vi "Digital_Bridge_3_kart.vi"() -> ()   [LabVIEW 2014] (continued)
                                n4059 = Index Array(array=w2316, index (row)=w2315, index (col)=w2314) -> (element=w2313:dbl)
                                n4060 = Replace Array Subset(array=w2316, new element=w2313, index (row)=w2315, index (col)=w2314) -> (w2317:dbl[][])
                                }
                                }
                                n4061 = local write "Denge Kosulu x2_y2"(w2257) -> ()
                                }
                              }
                              frame 3 {
                                n4062 = for {
                                N: 10 -> [_]
                                tunnel: w2318 -> [w2320]
                                i -> [w2323]
                                n4063 = local read "Denge Kosulu x2_y2"() -> (w2322:dbl[][])
                                n4064 = case shown="6" w2323 {
                                tunnel: w2323 -> [w2325 w2330 w2337 w2344 w2351 w2358 w2366 w2371 w2374 w2379]
                                tunnel: w2322 -> [w2326 w2332 w2336 w2343 w2350 w2357 w2364 w2369 w2375 w2380]
                                tunnel: [w2327 w2333 w2334 w2342 w2349 w2356 w2363 w2368 w2376 w2381] -> w2321
                                tunnel: w2320 -> [w2328 w2331 w2335 w2341 w2348 w2355 w2365 w2370 w2373 w2378]
                                frame 0, Default {
                                n4065 = Index Array(array=w2326, index (row)=w2325, index (col)=w2328) -> (element=w2324:dbl)
                                n4066 = Replace Array Subset(array=w2326, new element=w2324, index (row)=w2325, index (col)=w2328) -> (w2327:dbl[][])
                                }
                                frame 1 {
                                n4067 = Index Array(array=w2332, index (row)=w2330, index (col)=w2331) -> (element=w2329:dbl)
                                n4068 = Replace Array Subset(array=w2332, new element=w2329, index (row)=w2330, index (col)=w2331) -> (w2333:dbl[][])
                                }
                                frame 2 {
                                n4069 = Index Array(array=w2336, index (row)=w2337, index (col)=w2335) -> (element=w2340:dbl)
                                n4070 = Multiply(x=w2340, y=2.0) -> (x*y=w2338:dbl)
                                n4071 = Replace Array Subset(array=w2336, new element=w2338, index (row)=w2337, index (col)=w2335) -> (w2334:dbl[][])
                                }
                                frame 3 {
                                n4072 = Index Array(array=w2343, index (row)=w2344, index (col)=w2341) -> (element=w2347:dbl)
                                n4073 = Multiply(x=w2347, y=2.0) -> (x*y=w2345:dbl)
                                n4074 = Replace Array Subset(array=w2343, new element=w2345, index (row)=w2344, index (col)=w2341) -> (w2342:dbl[][])
                                }
                                frame 4 {
                                n4075 = Index Array(array=w2350, index (row)=w2351, index (col)=w2348) -> (element=w2354:dbl)
                                n4076 = Multiply(x=w2354, y=2.0) -> (x*y=w2352:dbl)
                                n4077 = Replace Array Subset(array=w2350, new element=w2352, index (row)=w2351, index (col)=w2348) -> (w2349:dbl[][])
                                }
                                frame 5 {
                                n4078 = Index Array(array=w2357, index (row)=w2358, index (col)=w2355) -> (element=w2361:dbl)
                                n4079 = Multiply(x=w2361, y=2.0) -> (x*y=w2359:dbl)
                                n4080 = Replace Array Subset(array=w2357, new element=w2359, index (row)=w2358, index (col)=w2355) -> (w2356:dbl[][])
                                }
                                frame 6 {
                                n4081 = Index Array(array=w2364, index (row)=w2366, index (col)=w2365) -> (element=w2362:dbl)
                                n4082 = Replace Array Subset(array=w2364, new element=w2362, index (row)=w2366, index (col)=w2365) -> (w2363:dbl[][])
                                }
                                frame 7 {
                                n4083 = Index Array(array=w2369, index (row)=w2371, index (col)=w2370) -> (element=w2367:dbl)
                                n4084 = Replace Array Subset(array=w2369, new element=w2367, index (row)=w2371, index (col)=w2370) -> (w2368:dbl[][])
                                }
                                frame 8 {
                                n4085 = Index Array(array=w2375, index (row)=w2374, index (col)=w2373) -> (element=w2372:dbl)
                                n4086 = Replace Array Subset(array=w2375, new element=w2372, index (row)=w2374, index (col)=w2373) -> (w2376:dbl[][])
                                }
                                frame 9 {
                                n4087 = Index Array(array=w2380, index (row)=w2379, index (col)=w2378) -> (element=w2377:dbl)
                                n4088 = Replace Array Subset(array=w2380, new element=w2377, index (row)=w2379, index (col)=w2378) -> (w2381:dbl[][])
                                }
                                }
                                n4089 = local write "Denge Kosulu x2_y2"(w2321) -> ()
                                }
                              }
                              frame 4, Default {
                                n4090 = for {
                                N: 10 -> [_]
                                tunnel: w2382 -> [w2384]
                                i -> [w2387]
                                n4091 = local read "Denge Kosulu x2_y2"() -> (w2386:dbl[][])
                                n4092 = case shown="6" w2387 {
                                tunnel: w2387 -> [w2389 w2394 w2402 w2407 w2412 w2417 w2421 w2428 w2434 w2439]
                                tunnel: w2386 -> [w2390 w2396 w2401 w2406 w2411 w2416 w2419 w2426 w2435 w2440]
                                tunnel: [w2391 w2397 w2399 w2405 w2410 w2415 w2418 w2425 w2436 w2441] -> w2385
                                tunnel: w2384 -> [w2392 w2395 w2400 w2404 w2409 w2414 w2420 w2427 w2433 w2438]
                                frame 0, Default {
                                n4093 = Index Array(array=w2390, index (row)=w2389, index (col)=w2392) -> (element=w2388:dbl)
                                n4094 = Replace Array Subset(array=w2390, new element=w2388, index (row)=w2389, index (col)=w2392) -> (w2391:dbl[][])
                                }
                                frame 1 {
                                n4095 = Index Array(array=w2396, index (row)=w2394, index (col)=w2395) -> (element=w2393:dbl)
                                n4096 = Replace Array Subset(array=w2396, new element=w2393, index (row)=w2394, index (col)=w2395) -> (w2397:dbl[][])
                                }
                                frame 2 {
                                n4097 = Index Array(array=w2401, index (row)=w2402, index (col)=w2400) -> (element=w2398:dbl)
                                n4098 = Replace Array Subset(array=w2401, new element=w2398, index (row)=w2402, index (col)=w2400) -> (w2399:dbl[][])
                                }
                                frame 3 {
                                n4099 = Index Array(array=w2406, index (row)=w2407, index (col)=w2404) -> (element=w2403:dbl)
                                n4100 = Replace Array Subset(array=w2406, new element=w2403, index (row)=w2407, index (col)=w2404) -> (w2405:dbl[][])
                                }
                                frame 4 {
                                n4101 = Index Array(array=w2411, index (row)=w2412, index (col)=w2409) -> (element=w2408:dbl)
                                n4102 = Replace Array Subset(array=w2411, new element=w2408, index (row)=w2412, index (col)=w2409) -> (w2410:dbl[][])
                                }
                                frame 5 {
                                n4103 = Index Array(array=w2416, index (row)=w2417, index (col)=w2414) -> (element=w2413:dbl)
                                n4104 = Replace Array Subset(array=w2416, new element=w2413, index (row)=w2417, index (col)=w2414) -> (w2415:dbl[][])
                                }
                                frame 6 {
                                n4105 = Index Array(array=w2419, index (row)=w2421, index (col)=w2420) -> (element=w2424:dbl)
                                n4106 = Multiply(x=w2424, y=2.0) -> (x*y=w2422:dbl)
                                n4107 = Replace Array Subset(array=w2419, new element=w2422, index (row)=w2421, index (col)=w2420) -> (w2418:dbl[][])
                                }
                                frame 7 {
                                n4108 = Index Array(array=w2426, index (row)=w2428, index (col)=w2427) -> (element=w2431:dbl)
                                n4109 = Multiply(x=w2431, y=2.0) -> (x*y=w2429:dbl)
                                n4110 = Replace Array Subset(array=w2426, new element=w2429, index (row)=w2428, index (col)=w2427) -> (w2425:dbl[][])
                                }
                                frame 8 {
                                n4111 = Index Array(array=w2435, index (row)=w2434, index (col)=w2433) -> (element=w2432:dbl)
                                n4112 = Replace Array Subset(array=w2435, new element=w2432, index (row)=w2434, index (col)=w2433) -> (w2436:dbl[][])
                                }
                                frame 9 {
                                n4113 = Index Array(array=w2440, index (row)=w2439, index (col)=w2438) -> (element=w2437:dbl)
                                n4114 = Replace Array Subset(array=w2440, new element=w2437, index (row)=w2439, index (col)=w2438) -> (w2441:dbl[][])
                                }
                                }
                                n4115 = local write "Denge Kosulu x2_y2"(w2385) -> ()
                                }
                              }
                              frame 5 {
                                n4116 = for {
                                N: 10 -> [_]
                                tunnel: w2442 -> [w2444]
                                i -> [w2447]
                                n4117 = local read "Denge Kosulu x2_y2"() -> (w2446:dbl[][])
                                n4118 = case shown="6" w2447 {
                                tunnel: w2447 -> [w2448 w2455 w2466 w2471 w2476 w2481 w2486 w2491 w2496 w2500]
                                tunnel: w2446 -> [w2449 w2457 w2465 w2470 w2475 w2480 w2484 w2489 w2497 w2501]
                                tunnel: [w2450 w2458 w2463 w2469 w2474 w2479 w2483 w2488 w2498 w2502] -> w2445
                                tunnel: w2444 -> [w2451 w2456 w2464 w2468 w2473 w2478 w2485 w2490 w2495 w2499]
                                frame 0, Default {
                                n4119 = Index Array(array=w2449, index (row)=w2448, index (col)=w2451) -> (element=w2454:dbl)
                                n4120 = Multiply(x=w2454, y=2.0) -> (x*y=w2452:dbl)
                                n4121 = Replace Array Subset(array=w2449, new element=w2452, index (row)=w2448, index (col)=w2451) -> (w2450:dbl[][])
                                }
                                frame 1 {
                                n4122 = Index Array(array=w2457, index (row)=w2455, index (col)=w2456) -> (element=w2461:dbl)
                                n4123 = Multiply(x=w2461, y=2.0) -> (x*y=w2459:dbl)
                                n4124 = Replace Array Subset(array=w2457, new element=w2459, index (row)=w2455, index (col)=w2456) -> (w2458:dbl[][])
                                }
                                frame 2 {
                                n4125 = Index Array(array=w2465, index (row)=w2466, index (col)=w2464) -> (element=w2462:dbl)
                                n4126 = Replace Array Subset(array=w2465, new element=w2462, index (row)=w2466, index (col)=w2464) -> (w2463:dbl[][])
                                }
                                frame 3 {
                                n4127 = Index Array(array=w2470, index (row)=w2471, index (col)=w2468) -> (element=w2467:dbl)
                                n4128 = Replace Array Subset(array=w2470, new element=w2467, index (row)=w2471, index (col)=w2468) -> (w2469:dbl[][])
                                }
                                frame 4 {
                                n4129 = Index Array(array=w2475, index (row)=w2476, index (col)=w2473) -> (element=w2472:dbl)
                                n4130 = Replace Array Subset(array=w2475, new element=w2472, index (row)=w2476, index (col)=w2473) -> (w2474:dbl[][])
                                }
                                frame 5 {
                                n4131 = Index Array(array=w2480, index (row)=w2481, index (col)=w2478) -> (element=w2477:dbl)
                                n4132 = Replace Array Subset(array=w2480, new element=w2477, index (row)=w2481, index (col)=w2478) -> (w2479:dbl[][])
                                }
                                frame 6 {
                                n4133 = Index Array(array=w2484, index (row)=w2486, index (col)=w2485) -> (element=w2482:dbl)
                                n4134 = Replace Array Subset(array=w2484, new element=w2482, index (row)=w2486, index (col)=w2485) -> (w2483:dbl[][])
                                }
                                frame 7 {
                                n4135 = Index Array(array=w2489, index (row)=w2491, index (col)=w2490) -> (element=w2487:dbl)
                                n4136 = Replace Array Subset(array=w2489, new element=w2487, index (row)=w2491, index (col)=w2490) -> (w2488:dbl[][])
                                }
                                frame 8 {
                                n4137 = Index Array(array=w2497, index (row)=w2496, index (col)=w2495) -> (element=w2494:dbl)
                                n4138 = Multiply(x=w2494, y=2.0) -> (x*y=w2492:dbl)
                                n4139 = Replace Array Subset(array=w2497, new element=w2492, index (row)=w2496, index (col)=w2495) -> (w2498:dbl[][])
                                }
                                frame 9 {
                                n4140 = Index Array(array=w2501, index (row)=w2500, index (col)=w2499) -> (element=w2505:dbl)
                                n4141 = Multiply(x=w2505, y=2.0) -> (x*y=w2503:dbl)
                                n4142 = Replace Array Subset(array=w2501, new element=w2503, index (row)=w2500, index (col)=w2499) -> (w2502:dbl[][])
                                }
                                }
                                n4143 = local write "Denge Kosulu x2_y2"(w2445) -> ()
                                }
                              }
                            }
                          }
                          frame #1 {
                            n4144 = local read "Denge Seçimi"() -> (w2507:u8)
                            n4145 = case shown="5" w2507 {
                              tunnel: w2506 -> [w2508 w2572 w2636 w2700 w2760]
                              frame 1 {
                                n4146 = for {
                                N: 10 -> [_]
                                tunnel: w2508 -> [w2510]
                                i -> [w2513]
                                n4147 = local read "Denge Kosulu x1_x2"() -> (w2512:dbl[][])
                                n4148 = case shown="0, Default" w2513 {
                                tunnel: w2513 -> [w2514 w2521 w2532 w2537 w2542 w2547 w2552 w2557 w2562 w2566]
                                tunnel: w2512 -> [w2515 w2523 w2531 w2536 w2541 w2546 w2550 w2555 w2563 w2567]
                                tunnel: [w2516 w2524 w2529 w2535 w2540 w2545 w2549 w2554 w2564 w2568] -> w2511
                                tunnel: w2510 -> [w2517 w2522 w2530 w2534 w2539 w2544 w2551 w2556 w2561 w2565]
                                frame 0, Default {
                                n4149 = Index Array(array=w2515, index (row)=w2514, index (col)=w2517) -> (element=w2520:dbl)
                                n4150 = Multiply(x=w2520, y=2.0) -> (x*y=w2518:dbl)
                                n4151 = Replace Array Subset(array=w2515, new element=w2518, index (row)=w2514, index (col)=w2517) -> (w2516:dbl[][])
                                }
                                frame 1 {
                                n4152 = Index Array(array=w2523, index (row)=w2521, index (col)=w2522) -> (element=w2527:dbl)
                                n4153 = Multiply(x=w2527, y=2.0) -> (x*y=w2525:dbl)
                                n4154 = Replace Array Subset(array=w2523, new element=w2525, index (row)=w2521, index (col)=w2522) -> (w2524:dbl[][])
                                }
                                frame 2 {
                                n4155 = Index Array(array=w2531, index (row)=w2532, index (col)=w2530) -> (element=w2528:dbl)
                                n4156 = Replace Array Subset(array=w2531, new element=w2528, index (row)=w2532, index (col)=w2530) -> (w2529:dbl[][])
                                }
                                frame 3 {
                                n4157 = Index Array(array=w2536, index (row)=w2537, index (col)=w2534) -> (element=w2533:dbl)
                                n4158 = Replace Array Subset(array=w2536, new element=w2533, index (row)=w2537, index (col)=w2534) -> (w2535:dbl[][])
                                }
                                frame 4 {
                                n4159 = Index Array(array=w2541, index (row)=w2542, index (col)=w2539) -> (element=w2538:dbl)
                                n4160 = Replace Array Subset(array=w2541, new element=w2538, index (row)=w2542, index (col)=w2539) -> (w2540:dbl[][])
                                }
                                frame 5 {
                                n4161 = Index Array(array=w2546, index (row)=w2547, index (col)=w2544) -> (element=w2543:dbl)
                                n4162 = Replace Array Subset(array=w2546, new element=w2543, index (row)=w2547, index (col)=w2544) -> (w2545:dbl[][])
                                }
                                frame 6 {
                                n4163 = Index Array(array=w2550, index (row)=w2552, index (col)=w2551) -> (element=w2548:dbl)
                                n4164 = Replace Array Subset(array=w2550, new element=w2548, index (row)=w2552, index (col)=w2551) -> (w2549:dbl[][])
                                }
                                frame 7 {
                                n4165 = Index Array(array=w2555, index (row)=w2557, index (col)=w2556) -> (element=w2553:dbl)
                                n4166 = Replace Array Subset(array=w2555, new element=w2553, index (row)=w2557, index (col)=w2556) -> (w2554:dbl[][])
                                }
                                frame 8 {
                                n4167 = Index Array(array=w2563, index (row)=w2562, index (col)=w2561) -> (element=w2560:dbl)
                                n4168 = Multiply(x=w2560, y=2.0) -> (x*y=w2558:dbl)
                                n4169 = Replace Array Subset(array=w2563, new element=w2558, index (row)=w2562, index (col)=w2561) -> (w2564:dbl[][])
                                }
                                frame 9 {
                                n4170 = Index Array(array=w2567, index (row)=w2566, index (col)=w2565) -> (element=w2571:dbl)
                                n4171 = Multiply(x=w2571, y=2.0) -> (x*y=w2569:dbl)
                                n4172 = Replace Array Subset(array=w2567, new element=w2569, index (row)=w2566, index (col)=w2565) -> (w2568:dbl[][])
                                }
                                }
                                n4173 = local write "Denge Kosulu x1_x2"(w2511) -> ()
                                }
                              }
                              frame 2 {
                                n4174 = for {
                                N: 10 -> [_]
                                tunnel: w2572 -> [w2574]
                                i -> [w2577]
                                n4175 = local read "Denge Kosulu x1_x2"() -> (w2576:dbl[][])
                                n4176 = case shown="0, Default" w2577 {
                                tunnel: w2577 -> [w2579 w2584 w2591 w2598 w2605 w2612 w2620 w2625 w2628 w2633]
                                tunnel: w2576 -> [w2580 w2586 w2590 w2597 w2604 w2611 w2618 w2623 w2629 w2634]
                                tunnel: [w2581 w2587 w2588 w2596 w2603 w2610 w2617 w2622 w2630 w2635] -> w2575
                                tunnel: w2574 -> [w2582 w2585 w2589 w2595 w2602 w2609 w2619 w2624 w2627 w2632]
                                frame 0, Default {
                                n4177 = Index Array(array=w2580, index (row)=w2579, index (col)=w2582) -> (element=w2578:dbl)
                                n4178 = Replace Array Subset(array=w2580, new element=w2578, index (row)=w2579, index (col)=w2582) -> (w2581:dbl[][])
                                }
                                frame 1 {
                                n4179 = Index Array(array=w2586, index (row)=w2584, index (col)=w2585) -> (element=w2583:dbl)
                                n4180 = Replace Array Subset(array=w2586, new element=w2583, index (row)=w2584, index (col)=w2585) -> (w2587:dbl[][])
                                }
                                frame 2 {
                                n4181 = Index Array(array=w2590, index (row)=w2591, index (col)=w2589) -> (element=w2594:dbl)
                                n4182 = Multiply(x=w2594, y=2.0) -> (x*y=w2592:dbl)
                                n4183 = Replace Array Subset(array=w2590, new element=w2592, index (row)=w2591, index (col)=w2589) -> (w2588:dbl[][])
                                }
                                frame 3 {
                                n4184 = Index Array(array=w2597, index (row)=w2598, index (col)=w2595) -> (element=w2601:dbl)
                                n4185 = Multiply(x=w2601, y=2.0) -> (x*y=w2599:dbl)
                                n4186 = Replace Array Subset(array=w2597, new element=w2599, index (row)=w2598, index (col)=w2595) -> (w2596:dbl[][])
                                }
                                frame 4 {
                                n4187 = Index Array(array=w2604, index (row)=w2605, index (col)=w2602) -> (element=w2608:dbl)
                                n4188 = Multiply(x=w2608, y=2.0) -> (x*y=w2606:dbl)
                                n4189 = Replace Array Subset(array=w2604, new element=w2606, index (row)=w2605, index (col)=w2602) -> (w2603:dbl[][])
                                }
                                frame 5 {
                                n4190 = Index Array(array=w2611, index (row)=w2612, index (col)=w2609) -> (element=w2615:dbl)
                                n4191 = Multiply(x=w2615, y=2.0) -> (x*y=w2613:dbl)
                                n4192 = Replace Array Subset(array=w2611, new element=w2613, index (row)=w2612, index (col)=w2609) -> (w2610:dbl[][])
                                }
                                frame 6 {
                                n4193 = Index Array(array=w2618, index (row)=w2620, index (col)=w2619) -> (element=w2616:dbl)
                                n4194 = Replace Array Subset(array=w2618, new element=w2616, index (row)=w2620, index (col)=w2619) -> (w2617:dbl[][])
                                }
                                frame 7 {
                                n4195 = Index Array(array=w2623, index (row)=w2625, index (col)=w2624) -> (element=w2621:dbl)
                                n4196 = Replace Array Subset(array=w2623, new element=w2621, index (row)=w2625, index (col)=w2624) -> (w2622:dbl[][])
                                }
                                frame 8 {
                                n4197 = Index Array(array=w2629, index (row)=w2628, index (col)=w2627) -> (element=w2626:dbl)
                                n4198 = Replace Array Subset(array=w2629, new element=w2626, index (row)=w2628, index (col)=w2627) -> (w2630:dbl[][])
                                }
                                frame 9 {
                                n4199 = Index Array(array=w2634, index (row)=w2633, index (col)=w2632) -> (element=w2631:dbl)
                                n4200 = Replace Array Subset(array=w2634, new element=w2631, index (row)=w2633, index (col)=w2632) -> (w2635:dbl[][])
                                }
                                }
                                n4201 = local write "Denge Kosulu x1_x2"(w2575) -> ()
                                }
                              }
                              frame 3 {
                                n4202 = for {
                                N: 10 -> [_]
                                tunnel: w2636 -> [w2638]
                                i -> [w2641]
                                n4203 = local read "Denge Kosulu x1_x2"() -> (w2640:dbl[][])
                                n4204 = case shown="0, Default" w2641 {
                                tunnel: w2641 -> [w2643 w2648 w2655 w2662 w2669 w2676 w2684 w2689 w2692 w2697]
                                tunnel: w2640 -> [w2644 w2650 w2654 w2661 w2668 w2675 w2682 w2687 w2693 w2698]
                                tunnel: [w2645 w2651 w2652 w2660 w2667 w2674 w2681 w2686 w2694 w2699] -> w2639
                                tunnel: w2638 -> [w2646 w2649 w2653 w2659 w2666 w2673 w2683 w2688 w2691 w2696]
                                frame 0, Default {
                                n4205 = Index Array(array=w2644, index (row)=w2643, index (col)=w2646) -> (element=w2642:dbl)
                                n4206 = Replace Array Subset(array=w2644, new element=w2642, index (row)=w2643, index (col)=w2646) -> (w2645:dbl[][])
                                }
                                frame 1 {
                                n4207 = Index Array(array=w2650, index (row)=w2648, index (col)=w2649) -> (element=w2647:dbl)
                                n4208 = Replace Array Subset(array=w2650, new element=w2647, index (row)=w2648, index (col)=w2649) -> (w2651:dbl[][])
                                }
                                frame 2 {
                                n4209 = Index Array(array=w2654, index (row)=w2655, index (col)=w2653) -> (element=w2658:dbl)
                                n4210 = Multiply(x=w2658, y=2.0) -> (x*y=w2656:dbl)
                                n4211 = Replace Array Subset(array=w2654, new element=w2656, index (row)=w2655, index (col)=w2653) -> (w2652:dbl[][])
                                }
                                frame 3 {
                                n4212 = Index Array(array=w2661, index (row)=w2662, index (col)=w2659) -> (element=w2665:dbl)
                                n4213 = Multiply(x=w2665, y=2.0) -> (x*y=w2663:dbl)
                                n4214 = Replace Array Subset(array=w2661, new element=w2663, index (row)=w2662, index (col)=w2659) -> (w2660:dbl[][])
                                }
                                frame 4 {
                                n4215 = Index Array(array=w2668, index (row)=w2669, index (col)=w2666) -> (element=w2672:dbl)
                                n4216 = Multiply(x=w2672, y=2.0) -> (x*y=w2670:dbl)
                                n4217 = Replace Array Subset(array=w2668, new element=w2670, index (row)=w2669, index (col)=w2666) -> (w2667:dbl[][])
                                }
                                frame 5 {
                                n4218 = Index Array(array=w2675, index (row)=w2676, index (col)=w2673) -> (element=w2679:dbl)
                                n4219 = Multiply(x=w2679, y=2.0) -> (x*y=w2677:dbl)
                                n4220 = Replace Array Subset(array=w2675, new element=w2677, index (row)=w2676, index (col)=w2673) -> (w2674:dbl[][])
                                }
                                frame 6 {
                                n4221 = Index Array(array=w2682, index (row)=w2684, index (col)=w2683) -> (element=w2680:dbl)
                                n4222 = Replace Array Subset(array=w2682, new element=w2680, index (row)=w2684, index (col)=w2683) -> (w2681:dbl[][])
                                }
                                frame 7 {
                                n4223 = Index Array(array=w2687, index (row)=w2689, index (col)=w2688) -> (element=w2685:dbl)
                                n4224 = Replace Array Subset(array=w2687, new element=w2685, index (row)=w2689, index (col)=w2688) -> (w2686:dbl[][])
                                }
                                frame 8 {
                                n4225 = Index Array(array=w2693, index (row)=w2692, index (col)=w2691) -> (element=w2690:dbl)
                                n4226 = Replace Array Subset(array=w2693, new element=w2690, index (row)=w2692, index (col)=w2691) -> (w2694:dbl[][])
                                }
                                frame 9 {
                                n4227 = Index Array(array=w2698, index (row)=w2697, index (col)=w2696) -> (element=w2695:dbl)
                                n4228 = Replace Array Subset(array=w2698, new element=w2695, index (row)=w2697, index (col)=w2696) -> (w2699:dbl[][])
                                }
                                }
                                n4229 = local write "Denge Kosulu x1_x2"(w2639) -> ()
                                }
                              }
                              frame 4, Default {
                                n4230 = for {
                                N: 10 -> [_]
                                tunnel: w2700 -> [w2702]
                                i -> [w2705]
                                n4231 = local read "Denge Kosulu x1_x2"() -> (w2704:dbl[][])
                                n4232 = case shown="0, Default" w2705 {
                                tunnel: w2705 -> [w2707 w2712 w2720 w2725 w2730 w2735 w2739 w2746 w2752 w2757]
                                tunnel: w2704 -> [w2708 w2714 w2719 w2724 w2729 w2734 w2737 w2744 w2753 w2758]
                                tunnel: [w2709 w2715 w2717 w2723 w2728 w2733 w2736 w2743 w2754 w2759] -> w2703
                                tunnel: w2702 -> [w2710 w2713 w2718 w2722 w2727 w2732 w2738 w2745 w2751 w2756]
                                frame 0, Default {
                                n4233 = Index Array(array=w2708, index (row)=w2707, index (col)=w2710) -> (element=w2706:dbl)
                                n4234 = Replace Array Subset(array=w2708, new element=w2706, index (row)=w2707, index (col)=w2710) -> (w2709:dbl[][])
                                }
                                frame 1 {
                                n4235 = Index Array(array=w2714, index (row)=w2712, index (col)=w2713) -> (element=w2711:dbl)
                                n4236 = Replace Array Subset(array=w2714, new element=w2711, index (row)=w2712, index (col)=w2713) -> (w2715:dbl[][])
                                }
                                frame 2 {
                                n4237 = Index Array(array=w2719, index (row)=w2720, index (col)=w2718) -> (element=w2716:dbl)
                                n4238 = Replace Array Subset(array=w2719, new element=w2716, index (row)=w2720, index (col)=w2718) -> (w2717:dbl[][])
                                }
                                frame 3 {
                                n4239 = Index Array(array=w2724, index (row)=w2725, index (col)=w2722) -> (element=w2721:dbl)
                                n4240 = Replace Array Subset(array=w2724, new element=w2721, index (row)=w2725, index (col)=w2722) -> (w2723:dbl[][])
                                }
                                frame 4 {
                                n4241 = Index Array(array=w2729, index (row)=w2730, index (col)=w2727) -> (element=w2726:dbl)
                                n4242 = Replace Array Subset(array=w2729, new element=w2726, index (row)=w2730, index (col)=w2727) -> (w2728:dbl[][])
                                }
                                frame 5 {
                                n4243 = Index Array(array=w2734, index (row)=w2735, index (col)=w2732) -> (element=w2731:dbl)
                                n4244 = Replace Array Subset(array=w2734, new element=w2731, index (row)=w2735, index (col)=w2732) -> (w2733:dbl[][])
                                }
                                frame 6 {
                                n4245 = Index Array(array=w2737, index (row)=w2739, index (col)=w2738) -> (element=w2742:dbl)
                                n4246 = Multiply(x=w2742, y=2.0) -> (x*y=w2740:dbl)
                                n4247 = Replace Array Subset(array=w2737, new element=w2740, index (row)=w2739, index (col)=w2738) -> (w2736:dbl[][])
                                }
                                frame 7 {
                                n4248 = Index Array(array=w2744, index (row)=w2746, index (col)=w2745) -> (element=w2749:dbl)
                                n4249 = Multiply(x=w2749, y=2.0) -> (x*y=w2747:dbl)
                                n4250 = Replace Array Subset(array=w2744, new element=w2747, index (row)=w2746, index (col)=w2745) -> (w2743:dbl[][])
                                }
                                frame 8 {
                                n4251 = Index Array(array=w2753, index (row)=w2752, index (col)=w2751) -> (element=w2750:dbl)
                                n4252 = Replace Array Subset(array=w2753, new element=w2750, index (row)=w2752, index (col)=w2751) -> (w2754:dbl[][])
                                }
                                frame 9 {
                                n4253 = Index Array(array=w2758, index (row)=w2757, index (col)=w2756) -> (element=w2755:dbl)
                                n4254 = Replace Array Subset(array=w2758, new element=w2755, index (row)=w2757, index (col)=w2756) -> (w2759:dbl[][])
                                }
                                }
                                n4255 = local write "Denge Kosulu x1_x2"(w2703) -> ()
                                }
                              }
                              frame 5 {
                                n4256 = for {
                                N: 10 -> [_]
                                tunnel: w2760 -> [w2762]
                                i -> [w2765]
                                n4257 = local read "Denge Kosulu x1_x2"() -> (w2764:dbl[][])
                                n4258 = case shown="9" w2765 {
                                tunnel: w2765 -> [w2766 w2773 w2784 w2789 w2794 w2799 w2804 w2809 w2814 w2818]
                                tunnel: w2764 -> [w2767 w2775 w2783 w2788 w2793 w2798 w2802 w2807 w2815 w2819]
                                tunnel: [w2768 w2776 w2781 w2787 w2792 w2797 w2801 w2806 w2816 w2820] -> w2763
                                tunnel: w2762 -> [w2769 w2774 w2782 w2786 w2791 w2796 w2803 w2808 w2813 w2817]
                                frame 0, Default {
                                n4259 = Index Array(array=w2767, index (row)=w2766, index (col)=w2769) -> (element=w2772:dbl)
                                n4260 = Multiply(x=w2772, y=2.0) -> (x*y=w2770:dbl)
                                n4261 = Replace Array Subset(array=w2767, new element=w2770, index (row)=w2766, index (col)=w2769) -> (w2768:dbl[][])
                                }
                                frame 1 {
                                n4262 = Index Array(array=w2775, index (row)=w2773, index (col)=w2774) -> (element=w2779:dbl)
                                n4263 = Multiply(x=w2779, y=2.0) -> (x*y=w2777:dbl)
                                n4264 = Replace Array Subset(array=w2775, new element=w2777, index (row)=w2773, index (col)=w2774) -> (w2776:dbl[][])
                                }
                                frame 2 {
                                n4265 = Index Array(array=w2783, index (row)=w2784, index (col)=w2782) -> (element=w2780:dbl)
                                n4266 = Replace Array Subset(array=w2783, new element=w2780, index (row)=w2784, index (col)=w2782) -> (w2781:dbl[][])
                                }
                                frame 3 {
                                n4267 = Index Array(array=w2788, index (row)=w2789, index (col)=w2786) -> (element=w2785:dbl)
                                n4268 = Replace Array Subset(array=w2788, new element=w2785, index (row)=w2789, index (col)=w2786) -> (w2787:dbl[][])
                                }
                                frame 4 {
                                n4269 = Index Array(array=w2793, index (row)=w2794, index (col)=w2791) -> (element=w2790:dbl)
                                n4270 = Replace Array Subset(array=w2793, new element=w2790, index (row)=w2794, index (col)=w2791) -> (w2792:dbl[][])
                                }
                                frame 5 {
                                n4271 = Index Array(array=w2798, index (row)=w2799, index (col)=w2796) -> (element=w2795:dbl)
                                n4272 = Replace Array Subset(array=w2798, new element=w2795, index (row)=w2799, index (col)=w2796) -> (w2797:dbl[][])
                                }
                                frame 6 {
                                n4273 = Index Array(array=w2802, index (row)=w2804, index (col)=w2803) -> (element=w2800:dbl)
                                n4274 = Replace Array Subset(array=w2802, new element=w2800, index (row)=w2804, index (col)=w2803) -> (w2801:dbl[][])
                                }
                                frame 7 {
                                n4275 = Index Array(array=w2807, index (row)=w2809, index (col)=w2808) -> (element=w2805:dbl)
                                n4276 = Replace Array Subset(array=w2807, new element=w2805, index (row)=w2809, index (col)=w2808) -> (w2806:dbl[][])
                                }
                                frame 8 {
                                n4277 = Index Array(array=w2815, index (row)=w2814, index (col)=w2813) -> (element=w2812:dbl)
                                n4278 = Multiply(x=w2812, y=2.0) -> (x*y=w2810:dbl)
                                n4279 = Replace Array Subset(array=w2815, new element=w2810, index (row)=w2814, index (col)=w2813) -> (w2816:dbl[][])
                                }
                                frame 9 {
                                n4280 = Index Array(array=w2819, index (row)=w2818, index (col)=w2817) -> (element=w2823:dbl)
                                n4281 = Multiply(x=w2823, y=2.0) -> (x*y=w2821:dbl)
                                n4282 = Replace Array Subset(array=w2819, new element=w2821, index (row)=w2818, index (col)=w2817) -> (w2820:dbl[][])
                                }
                                }
                                n4283 = local write "Denge Kosulu x1_x2"(w2763) -> ()
                                }
                              }
                            }
                          }
                          frame #2 {
                            n4284 = local read "Denge Seçimi"() -> (w2825:u8)
                            n4285 = case shown="2" w2825 {
                              tunnel: w2824 -> [w2826 w2890 w2954 w3018 w3078]
                              frame 1 {
                                n4286 = for {
                                N: 10 -> [_]
                                tunnel: w2826 -> [w2828]
                                i -> [w2831]
                                n4287 = local read "Denge Kosulu y1_y2"() -> (w2830:dbl[][])
                                n4288 = case shown="0, Default" w2831 {
                                tunnel: w2831 -> [w2832 w2839 w2850 w2855 w2860 w2865 w2870 w2875 w2880 w2884]
                                tunnel: w2830 -> [w2833 w2841 w2849 w2854 w2859 w2864 w2868 w2873 w2881 w2885]
                                tunnel: [w2834 w2842 w2847 w2853 w2858 w2863 w2867 w2872 w2882 w2886] -> w2829
                                tunnel: w2828 -> [w2835 w2840 w2848 w2852 w2857 w2862 w2869 w2874 w2879 w2883]
                                frame 0, Default {
                                n4289 = Index Array(array=w2833, index (row)=w2832, index (col)=w2835) -> (element=w2838:dbl)
                                n4290 = Multiply(x=w2838, y=2.0) -> (x*y=w2836:dbl)
                                n4291 = Replace Array Subset(array=w2833, new element=w2836, index (row)=w2832, index (col)=w2835) -> (w2834:dbl[][])
                                }
                                frame 1 {
                                n4292 = Index Array(array=w2841, index (row)=w2839, index (col)=w2840) -> (element=w2845:dbl)
                                n4293 = Multiply(x=w2845, y=2.0) -> (x*y=w2843:dbl)
                                n4294 = Replace Array Subset(array=w2841, new element=w2843, index (row)=w2839, index (col)=w2840) -> (w2842:dbl[][])
                                }
                                frame 2 {
                                n4295 = Index Array(array=w2849, index (row)=w2850, index (col)=w2848) -> (element=w2846:dbl)
                                n4296 = Replace Array Subset(array=w2849, new element=w2846, index (row)=w2850, index (col)=w2848) -> (w2847:dbl[][])
                                }
                                frame 3 {
                                n4297 = Index Array(array=w2854, index (row)=w2855, index (col)=w2852) -> (element=w2851:dbl)
                                n4298 = Replace Array Subset(array=w2854, new element=w2851, index (row)=w2855, index (col)=w2852) -> (w2853:dbl[][])
                                }
                                frame 4 {
                                n4299 = Index Array(array=w2859, index (row)=w2860, index (col)=w2857) -> (element=w2856:dbl)
                                n4300 = Replace Array Subset(array=w2859, new element=w2856, index (row)=w2860, index (col)=w2857) -> (w2858:dbl[][])
                                }
                                frame 5 {
                                n4301 = Index Array(array=w2864, index (row)=w2865, index (col)=w2862) -> (element=w2861:dbl)
                                n4302 = Replace Array Subset(array=w2864, new element=w2861, index (row)=w2865, index (col)=w2862) -> (w2863:dbl[][])
                                }
                                frame 6 {
                                n4303 = Index Array(array=w2868, index (row)=w2870, index (col)=w2869) -> (element=w2866:dbl)
                                n4304 = Replace Array Subset(array=w2868, new element=w2866, index (row)=w2870, index (col)=w2869) -> (w2867:dbl[][])
                                }
                                frame 7 {
                                n4305 = Index Array(array=w2873, index (row)=w2875, index (col)=w2874) -> (element=w2871:dbl)
                                n4306 = Replace Array Subset(array=w2873, new element=w2871, index (row)=w2875, index (col)=w2874) -> (w2872:dbl[][])
                                }
                                frame 8 {
                                n4307 = Index Array(array=w2881, index (row)=w2880, index (col)=w2879) -> (element=w2878:dbl)
                                n4308 = Multiply(x=w2878, y=2.0) -> (x*y=w2876:dbl)
                                n4309 = Replace Array Subset(array=w2881, new element=w2876, index (row)=w2880, index (col)=w2879) -> (w2882:dbl[][])
                                }
                                frame 9 {
                                n4310 = Index Array(array=w2885, index (row)=w2884, index (col)=w2883) -> (element=w2889:dbl)
                                n4311 = Multiply(x=w2889, y=2.0) -> (x*y=w2887:dbl)
                                n4312 = Replace Array Subset(array=w2885, new element=w2887, index (row)=w2884, index (col)=w2883) -> (w2886:dbl[][])
                                }
                                }
                                n4313 = local write "Denge Kosulu y1_y2"(w2829) -> ()
                                }
                              }
                              frame 2 {
                                n4314 = for {
                                N: 10 -> [_]
                                tunnel: w2890 -> [w2892]
                                i -> [w2895]
                                n4315 = local read "Denge Kosulu y1_y2"() -> (w2894:dbl[][])
                                n4316 = case shown="0, Default" w2895 {
                                tunnel: w2895 -> [w2897 w2902 w2909 w2916 w2923 w2930 w2938 w2943 w2946 w2951]
                                tunnel: w2894 -> [w2898 w2904 w2908 w2915 w2922 w2929 w2936 w2941 w2947 w2952]
                                tunnel: [w2899 w2905 w2906 w2914 w2921 w2928 w2935 w2940 w2948 w2953] -> w2893
                                tunnel: w2892 -> [w2900 w2903 w2907 w2913 w2920 w2927 w2937 w2942 w2945 w2950]
                                frame 0, Default {
                                n4317 = Index Array(array=w2898, index (row)=w2897, index (col)=w2900) -> (element=w2896:dbl)
                                n4318 = Replace Array Subset(array=w2898, new element=w2896, index (row)=w2897, index (col)=w2900) -> (w2899:dbl[][])
                                }
                                frame 1 {
                                n4319 = Index Array(array=w2904, index (row)=w2902, index (col)=w2903) -> (element=w2901:dbl)
                                n4320 = Replace Array Subset(array=w2904, new element=w2901, index (row)=w2902, index (col)=w2903) -> (w2905:dbl[][])
                                }
                                frame 2 {
                                n4321 = Index Array(array=w2908, index (row)=w2909, index (col)=w2907) -> (element=w2912:dbl)
                                n4322 = Multiply(x=w2912, y=2.0) -> (x*y=w2910:dbl)
                                n4323 = Replace Array Subset(array=w2908, new element=w2910, index (row)=w2909, index (col)=w2907) -> (w2906:dbl[][])
                                }
                                frame 3 {
                                n4324 = Index Array(array=w2915, index (row)=w2916, index (col)=w2913) -> (element=w2919:dbl)
                                n4325 = Multiply(x=w2919, y=2.0) -> (x*y=w2917:dbl)
                                n4326 = Replace Array Subset(array=w2915, new element=w2917, index (row)=w2916, index (col)=w2913) -> (w2914:dbl[][])
                                }
                                frame 4 {
                                n4327 = Index Array(array=w2922, index (row)=w2923, index (col)=w2920) -> (element=w2926:dbl)
                                n4328 = Multiply(x=w2926, y=2.0) -> (x*y=w2924:dbl)
                                n4329 = Replace Array Subset(array=w2922, new element=w2924, index (row)=w2923, index (col)=w2920) -> (w2921:dbl[][])
                                }
                                frame 5 {
                                n4330 = Index Array(array=w2929, index (row)=w2930, index (col)=w2927) -> (element=w2933:dbl)
                                n4331 = Multiply(x=w2933, y=2.0) -> (x*y=w2931:dbl)
                                n4332 = Replace Array Subset(array=w2929, new element=w2931, index (row)=w2930, index (col)=w2927) -> (w2928:dbl[][])
                                }
                                frame 6 {
                                n4333 = Index Array(array=w2936, index (row)=w2938, index (col)=w2937) -> (element=w2934:dbl)
                                n4334 = Replace Array Subset(array=w2936, new element=w2934, index (row)=w2938, index (col)=w2937) -> (w2935:dbl[][])
                                }
                                frame 7 {
                                n4335 = Index Array(array=w2941, index (row)=w2943, index (col)=w2942) -> (element=w2939:dbl)
                                n4336 = Replace Array Subset(array=w2941, new element=w2939, index (row)=w2943, index (col)=w2942) -> (w2940:dbl[][])
                                }
                                frame 8 {
                                n4337 = Index Array(array=w2947, index (row)=w2946, index (col)=w2945) -> (element=w2944:dbl)
                                n4338 = Replace Array Subset(array=w2947, new element=w2944, index (row)=w2946, index (col)=w2945) -> (w2948:dbl[][])
                                }
                                frame 9 {
                                n4339 = Index Array(array=w2952, index (row)=w2951, index (col)=w2950) -> (element=w2949:dbl)
                                n4340 = Replace Array Subset(array=w2952, new element=w2949, index (row)=w2951, index (col)=w2950) -> (w2953:dbl[][])
                                }
                                }
                                n4341 = local write "Denge Kosulu y1_y2"(w2893) -> ()
                                }
                              }
                              frame 3 {
                                n4342 = for {
                                N: 10 -> [_]
                                tunnel: w2954 -> [w2956]
                                i -> [w2959]
                                n4343 = local read "Denge Kosulu y1_y2"() -> (w2958:dbl[][])
                                n4344 = case shown="0, Default" w2959 {
                                tunnel: w2959 -> [w2961 w2966 w2973 w2980 w2987 w2994 w3002 w3007 w3010 w3015]
                                tunnel: w2958 -> [w2962 w2968 w2972 w2979 w2986 w2993 w3000 w3005 w3011 w3016]
                                tunnel: [w2963 w2969 w2970 w2978 w2985 w2992 w2999 w3004 w3012 w3017] -> w2957
                                tunnel: w2956 -> [w2964 w2967 w2971 w2977 w2984 w2991 w3001 w3006 w3009 w3014]
                                frame 0, Default {
                                n4345 = Index Array(array=w2962, index (row)=w2961, index (col)=w2964) -> (element=w2960:dbl)
                                n4346 = Replace Array Subset(array=w2962, new element=w2960, index (row)=w2961, index (col)=w2964) -> (w2963:dbl[][])
                                }
                                frame 1 {
                                n4347 = Index Array(array=w2968, index (row)=w2966, index (col)=w2967) -> (element=w2965:dbl)
                                n4348 = Replace Array Subset(array=w2968, new element=w2965, index (row)=w2966, index (col)=w2967) -> (w2969:dbl[][])
                                }
                                frame 2 {
                                n4349 = Index Array(array=w2972, index (row)=w2973, index (col)=w2971) -> (element=w2976:dbl)
                                n4350 = Multiply(x=w2976, y=2.0) -> (x*y=w2974:dbl)
                                n4351 = Replace Array Subset(array=w2972, new element=w2974, index (row)=w2973, index (col)=w2971) -> (w2970:dbl[][])
                                }
                                frame 3 {
                                n4352 = Index Array(array=w2979, index (row)=w2980, index (col)=w2977) -> (element=w2983:dbl)
                                n4353 = Multiply(x=w2983, y=2.0) -> (x*y=w2981:dbl)
                                n4354 = Replace Array Subset(array=w2979, new element=w2981, index (row)=w2980, index (col)=w2977) -> (w2978:dbl[][])
                                }
                                frame 4 {
                                n4355 = Index Array(array=w2986, index (row)=w2987, index (col)=w2984) -> (element=w2990:dbl)
                                n4356 = Multiply(x=w2990, y=2.0) -> (x*y=w2988:dbl)
                                n4357 = Replace Array Subset(array=w2986, new element=w2988, index (row)=w2987, index (col)=w2984) -> (w2985:dbl[][])
                                }
                                frame 5 {
                                n4358 = Index Array(array=w2993, index (row)=w2994, index (col)=w2991) -> (element=w2997:dbl)
                                n4359 = Multiply(x=w2997, y=2.0) -> (x*y=w2995:dbl)
                                n4360 = Replace Array Subset(array=w2993, new element=w2995, index (row)=w2994, index (col)=w2991) -> (w2992:dbl[][])
                                }
                                frame 6 {
                                n4361 = Index Array(array=w3000, index (row)=w3002, index (col)=w3001) -> (element=w2998:dbl)
                                n4362 = Replace Array Subset(array=w3000, new element=w2998, index (row)=w3002, index (col)=w3001) -> (w2999:dbl[][])
                                }
                                frame 7 {
                                n4363 = Index Array(array=w3005, index (row)=w3007, index (col)=w3006) -> (element=w3003:dbl)
                                n4364 = Replace Array Subset(array=w3005, new element=w3003, index (row)=w3007, index (col)=w3006) -> (w3004:dbl[][])
                                }
                                frame 8 {
                                n4365 = Index Array(array=w3011, index (row)=w3010, index (col)=w3009) -> (element=w3008:dbl)
                                n4366 = Replace Array Subset(array=w3011, new element=w3008, index (row)=w3010, index (col)=w3009) -> (w3012:dbl[][])
                                }
